vi "BasicOfQueues.vi"() -> ()   [LabVIEW 2020]
doc: "This VI demonstrates basic concepst of queues in LabVIEW. Comments in Polish."
panel:
  out "Error out":errorcluster
  out "Queue name":string
  out "Remaining elements":i32[](array[numeric])
  out "T_Out":bool caption="Timed out !"
  out "3":i32
  out "2":i32
  out "1":i32
  out "new2":bool caption="2 - created new?"
  out "new1":bool caption="1 created new?"
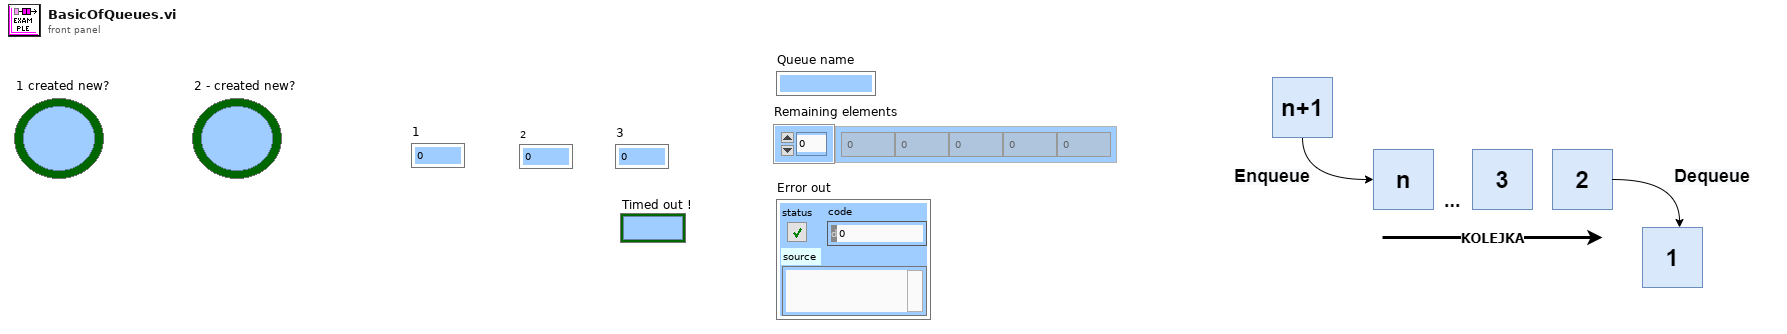
[diagram p1: front panel]
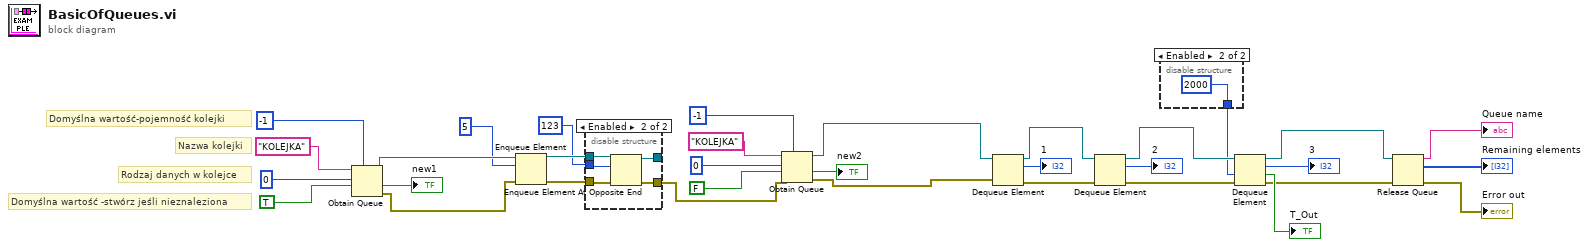
[diagram p0: block diagram]
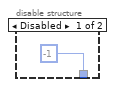
[diagram p2: hidden frame]
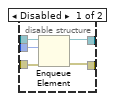
[diagram p3: hidden frame]
diagram:
  # "Rodzaj danych w kolejce"
  # "Nazwa kolejki"
  # "Domyślna wartość -stwórz jeśli nieznaleziona"
  # "Domyślna wartość-pojemność kolejki"
  n1 = Obtain Queue(max queue size (-1, unlimited)=-1, name (unnamed)="KOLEJKA", element data type=0, create if not found? (T)=TRUE) -> (queue out=w28:refnum<queue>, created new?=→"new1":bool, error out=w27:errorcluster)  [unwired: 1 in]
  n2 = Enqueue Element(queue=w28, element=5, error in (no error)=w27) -> (queue out=w24:refnum<queue>, error out=w25:errorcluster)  [unwired: 1 in, 1 out]
  n3 = disable-structure shown="Enabled" {
    disable-tunnel: w25 -> [w38 w42]
    disable-tunnel: w24 -> [w37 w43]
    disable-tunnel: 123 ("element") -> [w36 w39]
    disable-tunnel: [w34 w41] -> w20
    disable-tunnel: [w35 w40] -> _
    frame Disabled {
      n4 = Enqueue Element(queue=w37, element=w36, error in (no error)=w38) -> (queue out=w35:refnum<queue>, error out=w34:errorcluster)  [unwired: 1 in, 1 out]
    }
    frame Enabled {
      n5 = Enqueue Element At Opposite End(queue=w43, element=w39, error in (no error)=w42) -> (queue out=w40:refnum<queue>, error out=w41:errorcluster)  [unwired: 1 in, 1 out]
    }
  }
  n6 = Obtain Queue(max queue size (-1, unlimited)=-1, name (unnamed)="KOLEJKA", element data type=0, create if not found? (T)=FALSE, error in (no error)=w20) -> (queue out=w17:refnum<queue>, created new?=→"new2":bool, error out=w16:errorcluster)
  n7 = Dequeue Element(queue=w17, error in (no error)=w16) -> (queue out=w13:refnum<queue>, element=→"1":i32, error out=w12:errorcluster)  [unwired: 1 in, 1 out]
  n8 = Dequeue Element(queue=w13, error in (no error)=w12) -> (queue out=w9:refnum<queue>, element=→"2":i32, error out=w10:errorcluster)  [unwired: 1 in, 1 out]
  n9 = disable-structure shown="Enabled" {
    disable-tunnel: [-1 ("timeout in ms (-1)") 2000 ("timeout in ms (-1)")] -> w7
    frame Disabled {
    }
    frame Enabled {
    }
  }
  n10 = Dequeue Element(queue=w9, timeout in ms (-1)=w7, error in (no error)=w10) -> (queue out=w5:refnum<queue>, element=→"3":i32, timed out?=→"T_Out":bool, error out=w6:errorcluster)
  n11 = Release Queue(queue=w5, error in (no error)=w6) -> (queue name=→"Queue name":string, remaining elements=→"Remaining elements":i32[], error out=→"Error out":errorcluster)  [unwired: 1 in]
